vi "Read Windows1.vi"(8 "error in (no error)":errorcluster, 10 "win1 T:":bool, 11 "VISA resource name":refnum<visa-resource-name>) -> (0 "error out":errorcluster, 1 "offset past number":i32, 2 "read WIN1":string, 3 "VISA resource name out":refnum<visa-resource-name>, 4 "Blink T:":bool, 5 "read orgin":string)   [LabVIEW 2016]
panel:
  out "number":dbl
  in  "Timeout (10000 ms)":i32=10000 format="%#.6g"
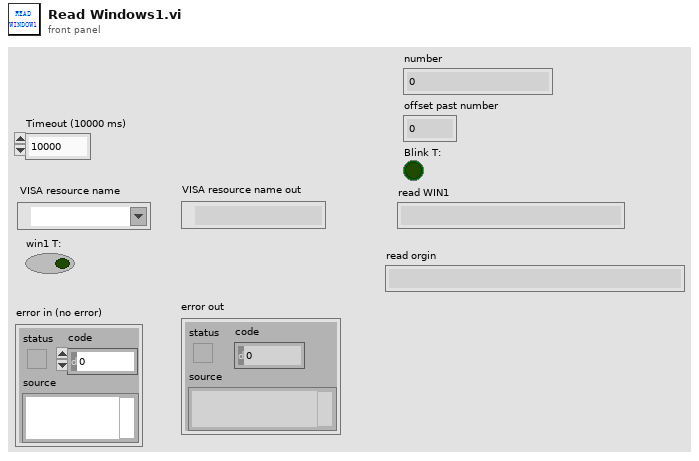
[diagram p1: front panel]
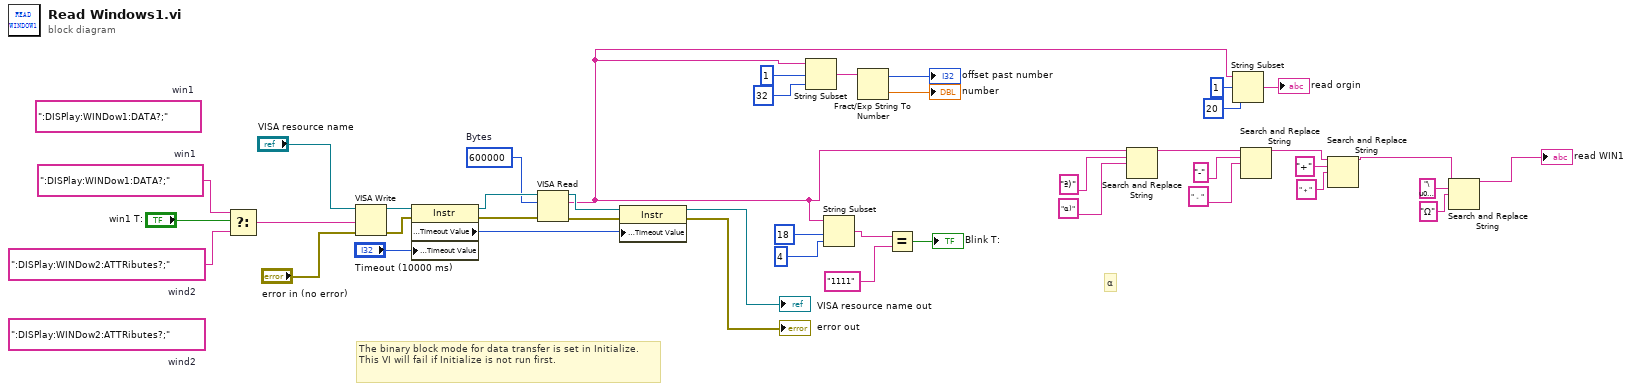
[diagram p0: block diagram]
diagram:
  (unwired) ":DISPlay:WINDow2:ATTRibutes?;"  # wind2
  (unwired) ":DISPlay:WINDow1:DATA?;"  # win1
  w25 = ":DISPlay:WINDow1:DATA?;"  # win1
  w24 = ":DISPlay:WINDow2:ATTRibutes?;"  # wind2
  w32 = u32 600000  # Bytes
  # "α"
  # "The binary block mode for data transfer is set in Initialize.  This VI will fail if Initialize is not run first."
  n1 = Select(t=w25, s="win1 T:", f=w24) -> (s? t:f=w22:string)
  n2 = VISA Write(VISA resource name="VISA resource name", write buffer=w22, error in (no error)="error in (no error)") -> (VISA resource name out=w31:refnum<visa-resource-name>, error out=w41:errorcluster)  [unwired: 1 out]
  n3 = property class="Instr"(reference=w31, error in=w41, "General Settings:Timeout Value"="Timeout (10000 ms)") -> (reference out=w40:refnum<visa-resource-name>, error out=w39:errorcluster, "General Settings:Timeout Value"=w35:u32)
  n4 = VISA Read(VISA resource name=w40, byte count=w32, error in (no error)=w39) -> (VISA resource name out=w37:refnum<visa-resource-name>, read buffer=w8:string, error out=w36:errorcluster)  [unwired: 1 out]
  n5 = property class="Instr"(reference=w37, error in=w36, "General Settings:Timeout Value"=w35) -> (reference out=→"VISA resource name out":refnum<visa-resource-name>, error out=→"error out":errorcluster)
  n6 = String Subset(string=w8, offset (0)=1, length (rest)=32 ("length (rest)")) -> (substring=w28:string)
  n7 = String Subset(string=w8, offset (0)=18, length (rest)=4 ("length (rest)")) -> (substring=w19:string)
  n8 = Fract/Exp String To Number(string=w28) -> (offset past number=→"offset past number":i32, number=→"number":dbl)  [unwired: 3 in]
  n9 = Equal?(x=w19, y="1111") -> (x = y?=→"Blink T:":bool)
  n10 = Search and Replace String(input string=w8, search string="ª)", replace string="α)" ("replace string (\"\")")) -> (result string=w9:string)  [unwired: 5 in, 3 out]
  n11 = String Subset(string=w8, offset (0)=1, length (rest)=20 ("length (rest)")) -> (substring=→"read orgin":string)
  n12 = Search and Replace String(input string=w9, search string="-", replace string="－" ("replace string (\"\")")) -> (result string=w12:string)  [unwired: 5 in, 3 out]
  n13 = Search and Replace String(input string=w12, search string="+", replace string="＋" ("replace string (\"\")")) -> (result string=w2:string)  [unwired: 5 in, 3 out]
  n14 = Search and Replace String(input string=w2, search string="\u0012", replace string="Ω" ("replace string (\"\")")) -> (result string=→"read WIN1":string)  [unwired: 5 in, 3 out]
